vi "tcp_connect_to_roborealm_final.vi"() -> (19 "error out gear tracking":errorcluster)   [LabVIEW 2017]
panel:
  in  "error in (no error) 4":errorcluster
  in  "error in (no error) 3":errorcluster
  in  "error in (no error) 2":errorcluster
  in  "error in (no error)":errorcluster
  out "error out fuel tracking":errorcluster
  in  "stop 3":bool
  in  "stop 1":bool
  in  "stop 2":bool
  out "error out boiler tracking":errorcluster
  out "error out peg tracking":errorcluster
  in  "stop":bool
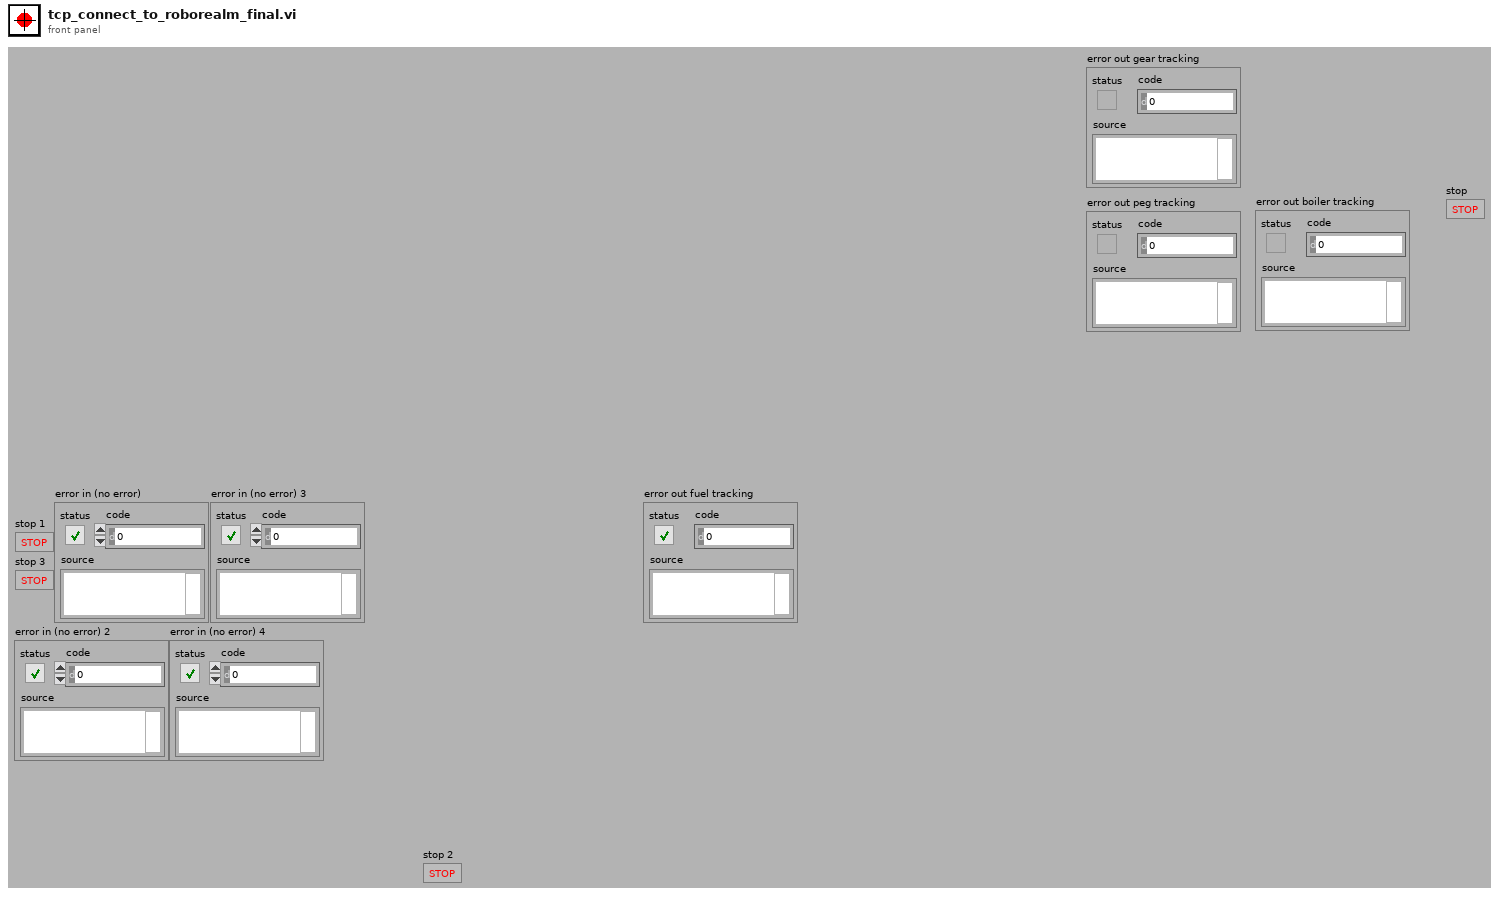
[diagram p1: front panel]
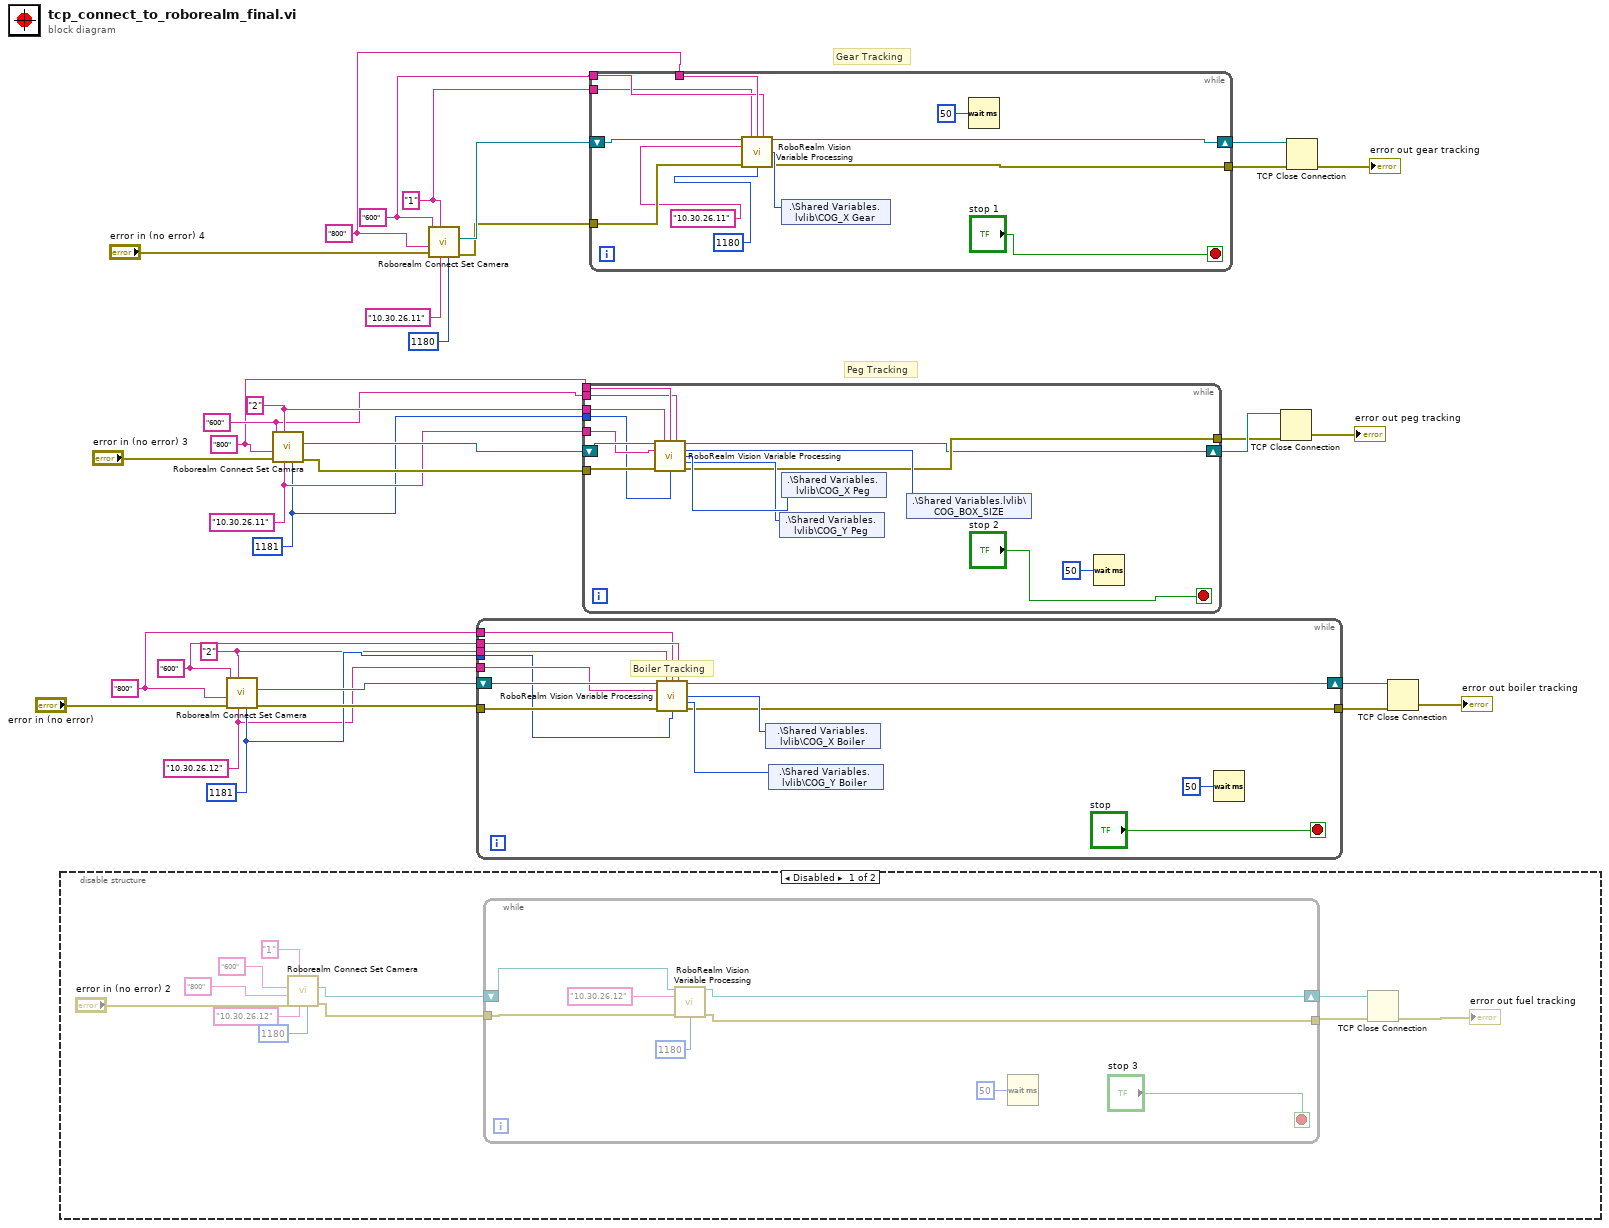
[diagram p0: block diagram]
diagram:
  w7 = "1" ("Camera")
  w6 = "600" ("Height")
  w5 = "800" ("Width")
  w15 = "2" ("Camera")
  w14 = "600" ("Height")
  w13 = "800" ("Width")
  w20 = u16 1181 ("remote port or service name")
  w19 = "10.30.26.12" ("address")
  w18 = "2" ("Camera")
  w17 = "600" ("Height")
  w16 = "800" ("Width")
  w23 = u16 1181 ("remote port or service name")
  w24 = "10.30.26.11" ("address")
  # "Gear Tracking"
  # "Peg Tracking"
  n1 = disable-structure shown="Disabled" {
    frame Disabled {
      n2 = call "Roborealm Connect Set Camera.vi"("remote port or service name"=u16 1180, "UP IP Address"="10.30.26.12", "Camera"="1", "error in (no error)"="error in (no error) 2", "Width"="800", "Height"="600") -> ("error out"=w41:errorcluster, "connection ID out"=w42:refnum<k5>)  [unwired: 4 in]
      n3 = while {
        tunnel: w41 -> [w52]
        tunnel: [w48] -> w36
        shift-right: [w47] -> w37
        shift-left: w42 -> [w50]
        stop <- "stop 3" stop-if-true
        n4 = call "RoboRealm Vision Variable Processing.vi"("connection ID in"=w50, "UP IP Address"="10.30.26.12", "error in"=w52, "remote port or service name"=u16 1180) -> ("connection ID out"=w47:refnum<k5>, "error out"=w48:errorcluster)  [unwired: 6 in, 4 out]
        n5 = Wait (ms)(milliseconds to wait=u32 50) -> ()  [unwired: 1 out]
      }
      n6 = TCP Close Connection(connection ID=w37, error in (no error)=w36) -> (error out=→"error out fuel tracking":errorcluster)  [unwired: 1 in, 1 out]
    }
    frame Enabled {
    }
  }
  n7 = call "Roborealm Connect Set Camera.vi"("remote port or service name"=w20, "UP IP Address"=w19, "Camera"=w15, "error in (no error)"="error in (no error)", "Width"=w13, "Height"=w14) -> ("error out"=w22:errorcluster, "connection ID out"=w21:refnum<k5>)  [unwired: 4 in]
  n8 = call "Roborealm Connect Set Camera.vi"("remote port or service name"=w23, "UP IP Address"=w24, "Camera"=w18, "error in (no error)"="error in (no error) 3", "Width"=w16, "Height"=w17) -> ("error out"=w25:errorcluster, "connection ID out"=w26:refnum<k5>)  [unwired: 4 in]
  n9 = call "Roborealm Connect Set Camera.vi"("remote port or service name"=u16 1180, "UP IP Address"="10.30.26.11" ("address"), "Camera"=w7, "error in (no error)"="error in (no error) 4", "Width"=w5, "Height"=w6) -> ("error out"=w9:errorcluster, "connection ID out"=w10:refnum<k5>)  [unwired: 4 in]
  n10 = while {
    tunnel: w22 -> [w64]
    tunnel: [w58] -> w28
    tunnel: w19 -> [w57]
    tunnel: w20 -> [w56]
    shift-right: [w59] -> w30
    shift-left: w21 -> [w65]
    tunnel: w15 -> [w55]
    tunnel: w14 -> [w54]
    tunnel: w13 -> [w53]
    stop <- "stop" stop-if-true
    # "Boiler Tracking"
    n11 = call "RoboRealm Vision Variable Processing.vi"("connection ID in"=w65, "Camera ID"=w55, "Image Width"=w53, "Image Height"=w54, "UP IP Address"=w57, "error in"=w64, "remote port or service name"=w56) -> ("connection ID out"=w59:refnum<k5>, "COG X"=w63:i32, "COG Y"=w62:i32, "error out"=w58:errorcluster)  [unwired: 3 in, 2 out]
    n12 = shared-variable ".\\Shared Variables.lvlib\\COG_X Boiler"(w63) -> ()  [unwired: 1 in, 1 out]
    n13 = shared-variable ".\\Shared Variables.lvlib\\COG_Y Boiler"(w62) -> ()  [unwired: 1 in, 1 out]
    n14 = Wait (ms)(milliseconds to wait=u32 50) -> ()  [unwired: 1 out]
  }
  n15 = while {
    tunnel: w25 -> [w78]
    tunnel: [w72] -> w27
    tunnel: w24 -> [w70]
    shift-right: [w71] -> w29
    shift-left: w26 -> [w79]
    tunnel: w23 -> [w69]
    tunnel: w18 -> [w68]
    tunnel: w17 -> [w66]
    tunnel: w16 -> [w67]
    stop <- "stop 2" stop-if-true
    n16 = call "RoboRealm Vision Variable Processing.vi"("connection ID in"=w79, "Camera ID"=w68, "Image Width"=w67, "Image Height"=w66, "UP IP Address"=w70, "error in"=w78, "remote port or service name"=w69) -> ("connection ID out"=w71:refnum<k5>, "COG_BOX_SIZE"=w75:i32, "COG X"=w77:i32, "COG Y"=w76:i32, "error out"=w72:errorcluster)  [unwired: 3 in, 1 out]
    n17 = shared-variable ".\\Shared Variables.lvlib\\COG_Y Peg"(w76) -> ()  [unwired: 1 in, 1 out]
    n18 = shared-variable ".\\Shared Variables.lvlib\\COG_X Peg"(w77) -> ()  [unwired: 1 in, 1 out]
    n19 = shared-variable ".\\Shared Variables.lvlib\\COG_BOX_SIZE"(w75) -> ()  [unwired: 1 in, 1 out]
    n20 = Wait (ms)(milliseconds to wait=u32 50) -> ()  [unwired: 1 out]
  }
  n21 = while {
    tunnel: w9 -> [w90]
    tunnel: [w86] -> w11
    shift-right: [w85] -> w12
    shift-left: w10 -> [w91]
    tunnel: w7 -> [w82]
    tunnel: w6 -> [w83]
    tunnel: w5 -> [w84]
    stop <- "stop 1" stop-if-true
    n22 = call "RoboRealm Vision Variable Processing.vi"("connection ID in"=w91, "Camera ID"=w82, "Image Width"=w84, "Image Height"=w83, "UP IP Address"="10.30.26.11" ("address"), "error in"=w90, "remote port or service name"=u16 1180) -> ("connection ID out"=w85:refnum<k5>, "COG X"=w89:i32, "error out"=w86:errorcluster)  [unwired: 3 in, 3 out]
    n23 = shared-variable ".\\Shared Variables.lvlib\\COG_X Gear"(w89) -> ()  [unwired: 1 in, 1 out]
    n24 = Wait (ms)(milliseconds to wait=u32 50) -> ()  [unwired: 1 out]
  }
  n25 = TCP Close Connection(connection ID=w29, error in (no error)=w27) -> (error out=→"error out peg tracking":errorcluster)  [unwired: 1 in, 1 out]
  n26 = TCP Close Connection(connection ID=w12, error in (no error)=w11) -> (error out=→"error out gear tracking":errorcluster)  [unwired: 1 in, 1 out]
  n27 = TCP Close Connection(connection ID=w30, error in (no error)=w28) -> (error out=→"error out boiler tracking":errorcluster)  [unwired: 1 in, 1 out]
